vi "RP Read IDN.vi"(6 "timeout ms (25000)":i32=500, 8 "Error In":errorcluster, 11 "connection ID":refnum<k5>) -> (0 "Error Out":errorcluster, 1 "Status response":u32=1 format="0x%x (%d)", 3 "connection ID out":refnum<k5>)   [LabVIEW 2015]
uses:
  RP Command.ctl
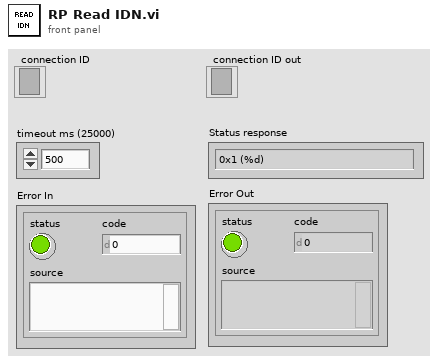
[diagram p1: front panel]
types:
  T1 = enum16{"big-endian, network order", "native, host order", "little-endian"}
  T2 = typedef "RP Command.ctl" = enum16{"Set frequency", "Read IDN", "Stop server", "Get status", "Get temperature", "Set decimation", "Arm", "Software trigger", "Get whole buffer", "Get chunk", "System call", "Get config", "Set config", "Read FIFO", "Play pattern", "Set frequency batch"}
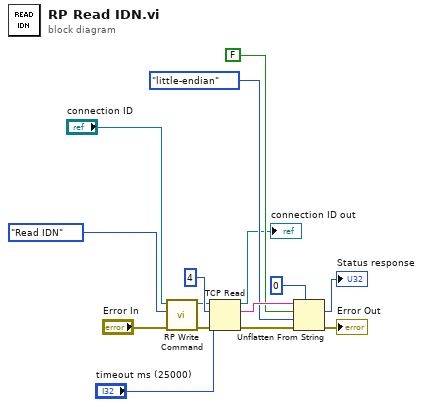
[diagram p0: block diagram]
diagram:
  n1 = call "RP Write Command.vi"("Error In"="Error In", "Command number"=RP_Command."Read IDN", "connection ID"="connection ID") -> ("Error Out"=w5:errorcluster, "connection ID out"=w6:refnum<k5>)  [unwired: 6 in, 1 out]
  n2 = TCP Read(connection ID=w6, bytes to read=4, error in (no error)=w5, 9:"timeout ms (25000)") -> (connection ID out=→"connection ID out":refnum<k5>, data out=w13:string, error out=w11:errorcluster)  [unwired: 1 in]
  n3 = Unflatten From String(type=u32 0, binary string=w13, data includes array or string size? (T)=FALSE, byte order (0:big-endian, network order)=T1."little-endian", error in (no error)=w11) -> (value=→"Status response":u32, error out=→"Error Out":errorcluster)  [unwired: 1 out]
